vi "SetFullName.vi"(8 "error in (no error)":errorcluster, 10 "FileName":string, 11 "DocumentClass in":refnum<class "Characteristic.lvclass">) -> (0 "error out":errorcluster, 3 "DocumentClass out":refnum<class "Characteristic.lvclass">)   [LabVIEW 2021, in "ProligentXMLGenerator.lvlib" / "Characteristic.lvclass"]
doc: "Set Full Name\n\nCharacteristics are unique among siblings by their FullName property.\n\nIt's limited to 434 characters."
uses:
  Characteristic.lvclass
  Characteristic.lvclass/Characteristic.ctl
  Base/NonEmptyString_434/NonEmptyString_434.lvclass
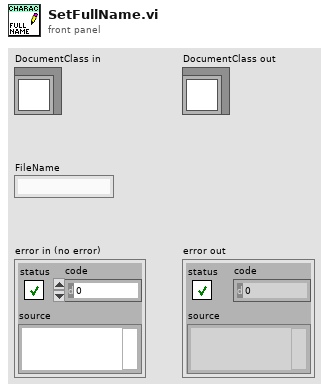
[diagram p1: front panel]
types:
  T1 = typedef "ProligentXMLGenerator.lvlib/Characteristic.lvclass/Data.ctl" = cluster{"Name":string, "CustomData":refnum<class "CustomData.lvclass">, "FullName":refnum<class "NonEmptyString_434.lvclass">, "Value":refnum<class "String_2000.lvclass">}
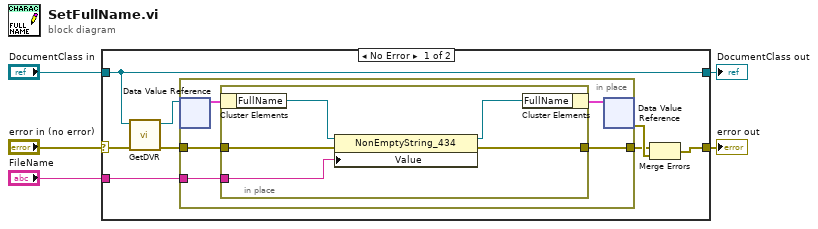
[diagram p0: block diagram]
diagram:
  n1 = case shown="No Error" "error in (no error)" {
    selector: "error in (no error)" -> [w11 w24]
    tunnel: "DocumentClass in" -> [w6 w25]
    tunnel: [w8 w24] -> w2
    tunnel: "FileName" -> [w7 _]
    tunnel: [w6 w25] -> w4
    frame No Error {
      n2 = call "GetDVR.vi"("error in"=w11, "Document in"=w6) -> ("error out"=w10:errorcluster, "DVRReference"=w12:refnum<data-value>)  [unwired: 8 in]
      n3 = in-place "In Place Element Structure" {
        in-place-border: w10 -> [w18]
        in-place-border: [w17] -> w9
        in-place-border: w7 -> [w16]
        n4 = in-place-dvr #1(w12) -> (w15:T1)  [unwired: 1 out]
        n5 = in-place "In Place Element Structure" {
          in-place-border: w18 -> [w23]
          in-place-border: [w22] -> w17
          in-place-border: w16 -> [w21]
          n6 = in-place-cluster #2(w15) -> ("FullName"=w20:refnum<class "NonEmptyString_434.lvclass">)
          n7 = property on="Property Node" class="NonEmptyString_434"(reference=w20, error in=w23, "Value"=w21) -> (reference out=w19:refnum<class "NonEmptyString_434.lvclass">, error out=w22:errorcluster)
          n8 = in-place-cluster #2("FullName"=w19) -> (w14:T1)
        }
        n9 = in-place-dvr #1(w14) -> (w13:errorcluster)  [unwired: 1 out]
      }
      n10 = Merge Errors(w9, w13) -> (w8:errorcluster)
    }
    frame Error {
    }
  }
  "error out" <- w2
  "DocumentClass out" <- w4
